vi "Open Remote uService GUI.vi"(8 "error in (no error)":errorcluster, 9 "GUI VI":refnum<vi>, 10 "uService ID":string, 11 "Message Enqueuer":refnum<class "Common GUI v3.lvclass">) -> (0 "error out":errorcluster, 1 "Remote GUI ref":refnum<vi>, 2 "uService ID dup":string)   [LabVIEW 2026, in "TALOS.lvlib" / "Common GUI v3.lvlib"]
uses:
  Common GUI v3.lvlib
  Common GUI v3/Common GUI v3.lvclass
  Remote uService GUI.vi
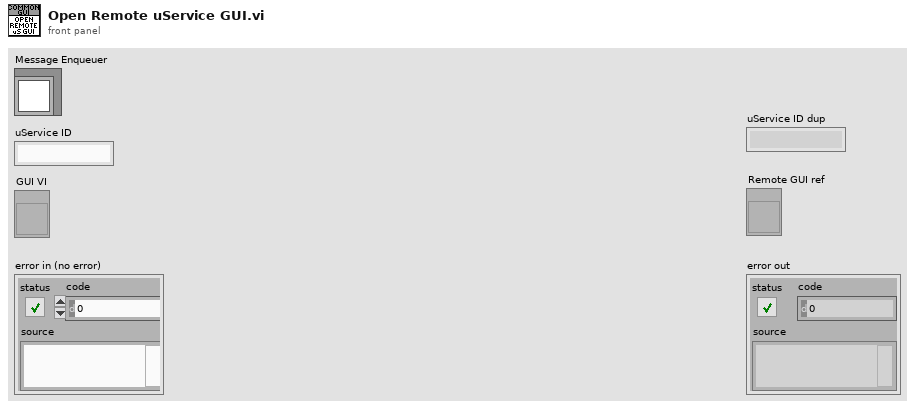
[diagram p1: front panel]
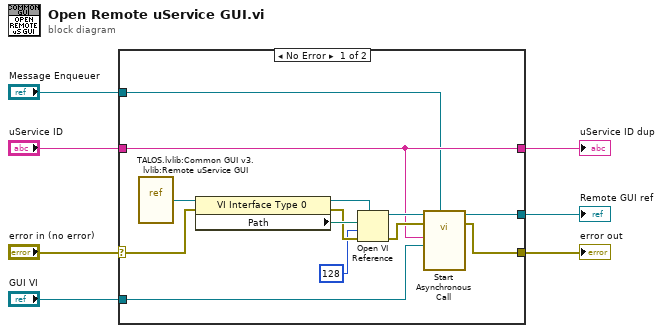
[diagram p0: block diagram]
diagram:
  n1 = case shown="No Error" "error in (no error)" {
    selector: "error in (no error)" -> [w16 w22]
    tunnel: "GUI VI" -> [w12 _]
    tunnel: "uService ID" -> [w9 w21]
    tunnel: "Message Enqueuer" -> [w8 _]
    tunnel: [w11 _] -> w3
    tunnel: [w10 w22] -> w2
    tunnel: [w9 w21] -> w1
    frame No Error {
      n2 = vi-ref "TALOS.lvlib:Common GUI v3.lvlib:Remote uService GUI.vi"() -> (w20:refnum<vi>)
      n3 = property class="VI Interface Type 0"(reference=w20, error in=w16) -> (reference out=w18:refnum<vi>, error out=w17:errorcluster, "Path"=w19:path)
      n4 = Open VI Reference(type specifier VI Refnum (for type only)=w18, vi path=w19, options=128, error in (no error)=w17) -> (vi reference=w14:refnum<vi>, error out=w13:errorcluster)  [unwired: 2 in]
      n5 = call-by-ref "Start Asynchronous Call"(reference=w14, error in=w13, "Message Enqueuer"=w8, "GUI VI"=w12, "uService ID"=w9) -> (reference out=w11:refnum<vi>, error out=w10:errorcluster)  [unwired: 9 in]
    }
    frame Error {
    }
  }
  "Remote GUI ref" <- w3
  "error out" <- w2
  "uService ID dup" <- w1
